vi "ASE Kalman_Experiment_FPGA.vi"() -> ()   [LabVIEW 2018]
doc: "This example demonstrates a simple analog loopback."
uses:
  <vilib>/Simulation/Scripting/Companion Diagram/SimConfigNode/SimDog.xnode
  <vilib>/Simulation/Implementation/Shared/SIMSCR Execution Mode.ctl
  <vilib>/Simulation/Scripting/Companion Diagram/SimConfigNode/_simSolvers.ctl
  <vilib>/Simulation/Scripting/Companion Diagram/SimConfigNode/SimParams.ctl
  <vilib>/Simulation/Implementation/XNodeFramework/SimXNode/SimX.xnode
  <vilib>/Simulation/SignalArithmetic/Implementation/NILVSim Gain.llb/SIM Gain (scalar).vi
  <vilib>/Simulation/ContinuousLinear/Implementation/NILVSim Transfer Function.llb/SIM Transfer Function (SISO).vi
  <vilib>/Simulation/Utility/Implementation/SIM Halt.vi
  <vilib>/Simulation/DataSources/Implementation/NILVSim Signal Generator.llb/SIM Signal Generator (scalar).vi
  <vilib>/Simulation/Nonlinear/Implementation/NILVSim Saturation.llb/SIM Saturation (scalar).vi
  <vilib>/Simulation/Nonlinear/Implementation/NILVSim RateLimiter.llb/SIM RateLimiter (scalar).vi
  <vilib>/Simulation/ContinuousLinear/Implementation/NILVSim Integrator new.llb/SIM Integrator (scalar).vi
  <vilib>/rvi/interface/nirviReadWriteControl/nirviReadWriteControl.xnode
  NiFpgaLv.dll
  <vilib>/Utility/error.llb/Error Cluster From Error Code.vi
  <vilib>/rvi/interface/Simulation/niFpgaSimulationCallBeginRW.vi
  <vilib>/rvi/errors/niLvFpgaAdjustHostInterfaceError.vi
  <vilib>/Quanser/Rapid Control Prototyping Toolkit/discrete/CL Bias Removal.vi
  <vilib>/Quanser/Rapid Control Prototyping Toolkit/discrete/_TypeSpecific/CL Bias Removal (Scalar).vi
  <vilib>/rvi/interface/nirviOpenFPGA/nirviOpenFPGA.xnode
  <vilib>/Simulation/SignalArithmetic/Implementation/NILVSim Gain.llb/SIM Gain (vector).vi
  <vilib>/Simulation/Nonlinear/Implementation/NILVSim Saturation.llb/SIM Saturation (vector).vi
  <vilib>/rvi/interface/nirviCloseFPGA/nirviCloseFPGA.xnode
  <vilib>/FPGAPlugInAG/Dynamic/niLvFpga_Close_Dynamic.vi
  <vilib>/addons/Control Design/_Stochastic Systems/NI_CD_Stochastic Systems.lvlib
  <vilib>/addons/Control Design/_Stochastic Systems/Stochastic Systems.llb/CD Construct Stochastic Model (Numeric).vi
  <vilib>/addons/Control Design/_Stochastic Systems/Stochastic Systems.llb/CD Construct Noise Model (Numeric).vi
  <vilib>/addons/Control Design/_Implementation/CD Continuous Recursive Kalman Filter.vi
  <vilib>/imath/engines/lvmath2/RunTimeEngine/Managers/WorkSpace/UID Generator.vi
  <vilib>/imath/engines/lvmath2/RunTimeEngine/LocalVariableDefStatement/MC_LocalVariableDefStatement_Display.vi
  <vilib>/imath/engines/lvmath2/RunTimeEngine/RunTimeType/NIMS_RunTimeType_From StrictType (excl LVString).vi
  <vilib>/imath/engines/lvmath2/RunTimeEngine/Managers/SymbolTable/Clear UID.vi
  <vilib>/imath/engines/lvmath2/RunTimeEngine/Managers/SymbolTable/NIMS_WorkSpace.lvlib
  <vilib>/imath/engines/lvmath2/RunTimeEngine/NodeEndStatement/NIMS_NodeEndStatement_Output.vi
  <vilib>/imath/engines/lvmath2/RunTimeEngine/ErrorHandling/NIMS_Finalize Error.vi
  <vilib>/Simulation/SignalDisplay/Implementation/NILVSim Time Waveform.llb/SIM Time Waveform (vector).vi
  FPGA Bitfiles/ActiveSuspension_FPGATarget_FPGAQ1MODULE_-QPaFzs6Ihw.lvbitx
  FPGA_Q1_MODULE.vi
  <vilib>/FPGAPlugInAG/cRIO-9068/niLvFpga_Open_cRIO-9068.vi
  <vilib>/rvi/interface/common/dynamic/niFpgaDynamicAddResources.vi
panel:
  out "Kalman Filter":waveform(dbl)[](graph)=[{"t0"=timestamp(9.964 s since 1904-01-01), "dt"=1.0, "Y"=[0.009999999999999988]}, {"t0"=timestamp(9.964 s since 1904-01-01), "dt"=1.0, "Y"=[0.008101035650175014]}, {"t0"=timestamp(9.964 s since 1904-01-01), "dt"=1.0, "Y"=[0.0033426903430059957]}]
  out "Measured value":T1(graph)={"output"=0.0096065956, "Result"=0.0090666584, "output"=0.0091514816}
  in  "R":dbl[][](array[numeric])=[[0.001, 0.0], [0.0, 0.001]] format="%#.5f"
  in  "Q":dbl[][](array[numeric])=[[0.001, 0.0, 0.0, 0.0], [0.0, 0.001, 0.0, 0.0], [0.0, 0.0, 0.001, 0.0], [0.0, 0.0, 0.0, 0.001]] format="%#.4f"
  in  "Enable Motor":bool
  in  "Setpoint Command":T2={"Amplitude (m)"=0.01, "Frequency (Hz)"=0.3} caption="Road (Bottom Plate)\nAmplitude Command (m)" {"Frequency (Hz)" min=0.0 max=0.5 step=0.009999999776482582 format="%_3f"; "Amplitude (m)" min=-10.0 max=10.0 step=0.5 format="%_3f"}
  in  "Halt?":bool
  # "Active Suspension Adaptive Control Experiment"
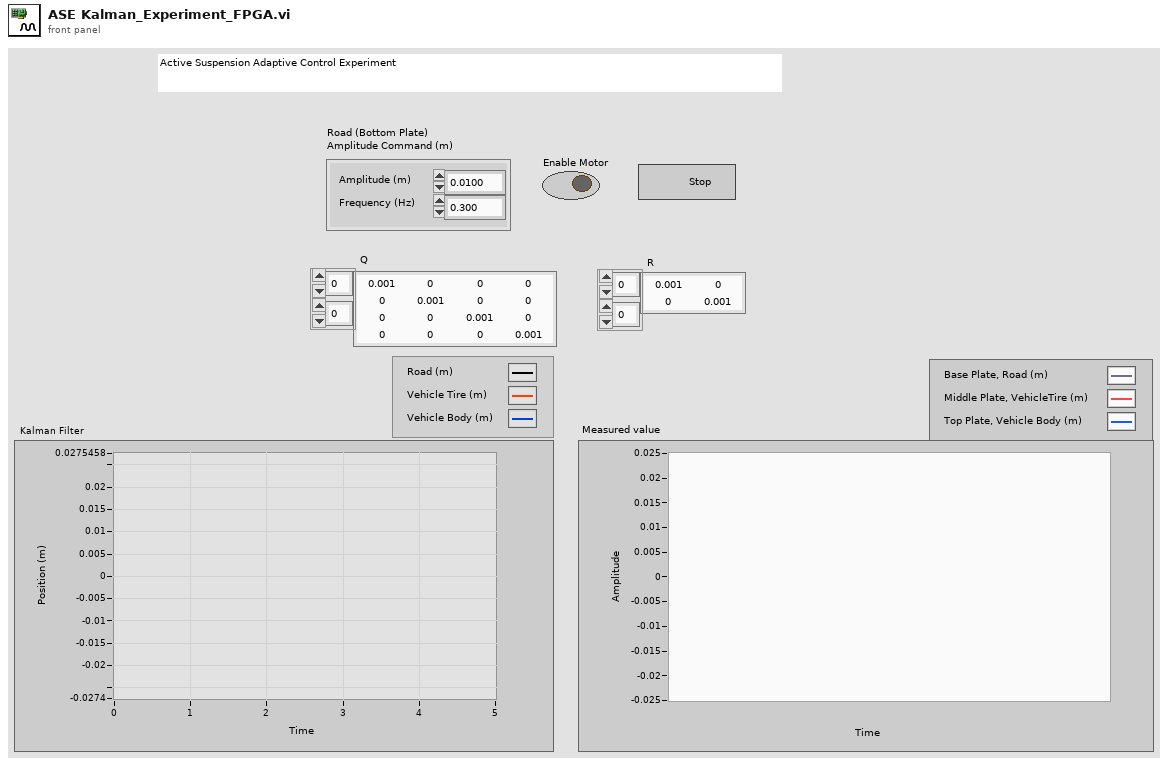
[diagram p1: front panel]
types:
  T1 = cluster{"output":dbl, "Result":dbl, "output":dbl}
  T2 = cluster{"Amplitude (m)":dbl, "Frequency (Hz)":dbl}
  T3 = typedef "SimParams.ctl" = cluster{"Initial Time (s)":dbl, "Final Time (s)":dbl, "Step Size (s)":dbl, "ODE Solver":T4, "Minimum Step Size (s)":dbl, "Maximum Step Size (s)":dbl, "Relative Tolerance":dbl, "Absolute Tolerance":dbl, "Software Timing":bool, "Initial Step Size (s)":dbl, "Automatic Fixed Step Size?":bool, "Automatic Discrete Step Size?":bool, "Discrete Step Size (s)":dbl, "Calculate using Time Step":bool, "Solver Wired?":bool, "Prev.Frm.Expected End":u64, "Prev.Frm.Actual End":u64, "Prev.Frm.Finished Late?":bool, "Prev.Iter.Expected End":u64, "Prev.Iter.Actual End":u64, "Prev.Iter.Finished Late?":bool, "Expected Iteration Start":u64, "Actual Iteration Start":u64, "Expected Frame Start":u64, "Actual Frame Start":u64, "Source Name":string, "Name":string, "Period":i64, "Deadline":i64, "Offset":i64, "Start":i64, "Priority":i32, "Timeout":i32, "Processor":i32, "Mode":enum32{"No Change", "Process missed periods, maintain original phase", "Discard missed periods, maintain original phase", "Process missed periods, ignore original phase", "Discard missed periods, ignore original phase"}, "Wakeup reason":enum32{"Normal", "Aborted", "Asynchronous wakeup", "Timing source error", "Timed loop error", "Timeout"}, "Error":errorcluster, "Source Type":string, "Secondary Source Type":string, "Global End Time":u64, "Global Start Time":u64, "Full Solver Reset":bool, "Execution Mode":T5, "Nan/Inf Check":bool, "Custom Solver Library":string, "Solver Is Variable":bool, "custom solver name":string, "Signal Collection Decimation":u32}
  T4 = typedef "_simSolvers.ctl" = enum16{"Runge-Kutta 1 (Euler)", "Runge-Kutta 2", "Runge-Kutta 3", "Runge-Kutta 4", "Runge-Kutta 23 (variable)", "Runge-Kutta 45 (variable)", "BDF (variable)", "Adams-Moulton (variable)", "Rosenbrock (variable)", "Discrete States Only", "SDIRK 4 (variable)", "Radau 5 (variable)", "Radau 9 (variable)", "Radau 13 (variable)", "Radau [Variable Order] (variable)", "Gear's Method (variable)", "Linearizer", "State Query", "Trim Eval", "Custom Solver"}
  T5 = typedef "SIMSCR Execution Mode.ctl" = enum16{"Simulate to Completion", "Single Time-Step Simulation (Fixed Step Only)"}
  T6 = typedef "NI_CD_Stochastic Systems.lvlib/cd_Stochastic State-Space Model.ctl" = cluster{"Sampling Time (s)":dbl, "G":dbl[][], "B":dbl[][], "A":dbl[][], "C":dbl[][], "D":dbl[][], "H":dbl[][]}
  T7 = typedef "NI_CD_Stochastic Systems.lvlib/cd_Second-Order Statistics Noise Model.ctl" = cluster{"Q":dbl[][], "E{w}":dbl[], "E{v}":dbl[], "R":dbl[][], "N":dbl[][]}
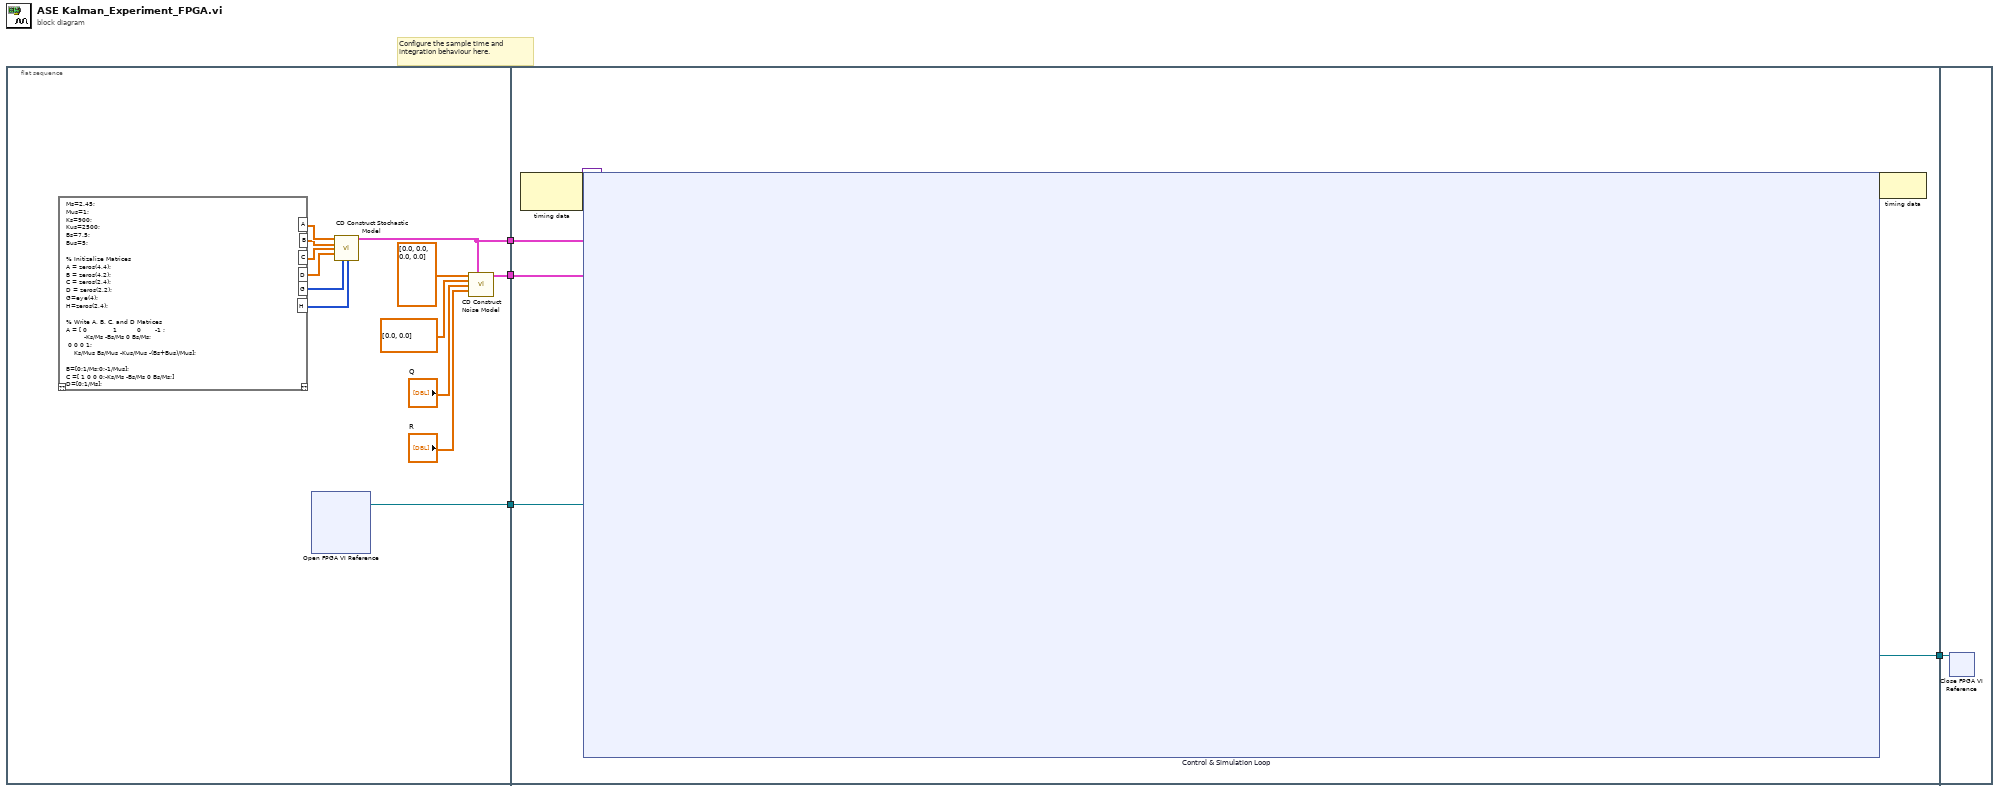
[diagram p0: block diagram]
diagram:
  # "Configure the sample time and integration behaviour here."
  n1 = flat-sequence {
    tunnel: [w17] -> w4
    tunnel: [w6] -> w2
    tunnel: [w5] -> w1
    tunnel: w4 -> [w207]
    tunnel: [w208] -> w3
    tunnel: w2 -> [w206]
    tunnel: w1 -> [w205]
    tunnel: w3 -> [w445]
    frame #0 {
      n2 = mathscript code="Ms=2.45;\nMus=1;\nKs=900;\nKus=2500;\nBs=7.5;\nBus=5;\n\n% Initizalize Matrices\nA = zeros(4,4);\nB = zeros(4,2);\nC = zeros(2,4);\nD = zeros(2,2);\nG=eye(4);\nH=zeros(2,4);\n\n% Write A, B, C, and D Matrices\nA = [ 0             1          0       -1 ; \n         -Ks/Ms -Bs/Ms 0 Bs/Ms;  \n 0 0 0 1;\n    Ks/Mus Bs/Mus -Kus/Mus -(Bs+Bus)/Mus];\n\nB=[0;1/Ms;0;-1/Mus];\nC =[ 1 0 0 0;-Ks/Ms -Bs/Ms 0 Bs/Ms;]\nD=[0;1/Ms];"() -> ("A"=w16:dbl[][], "B"=w14:dbl[][], "C"=w15:dbl[][], "D"=w13:dbl[][], "G"=w10:i32[][], "H"=w9:i32[][])  [unwired: 1 in, 1 out]
      n3 = xnode "Open FPGA VI Reference"() -> ("FPGA VI Reference Out"=w17:refnum<k20>)  [unwired: 2 in, 1 out]
      n4 = call-poly <vilib>:"CD Construct Stochastic Model.vi"("A"=w16, "B"=w14, "C"=w15, "D"=w13, "G"=w10, "H"=w9) -> ("Stochastic State-Space Model"=w6:T6)  [unwired: 2 in, 7 out]
      n5 = call-poly <vilib>:"CD Construct Noise Model.vi"("E{w}"=dbl[] [0.0, 0.0, 0.0, 0.0], "Stochastic State-Space Model"=w6, "E{v}"=dbl[] [0.0, 0.0], "Q"="Q", "R"="R") -> ("Second-Order Statistics Noise Model out"=w5:T7)  [unwired: 9 in, 1 out]
    }
    frame #1 {
      n6 = node-c288() -> (w210:variant)  [unwired: 2 in]
      n7 = node-c254 "Control & Simulation Loop"(w210, w207, w206, w205) -> (w209:variant, w208:refnum<k20>)
      n8 = node-c288(w209) -> ()  [unwired: 1 out]
    }
    frame #2 {
      n9 = xnode "Close FPGA VI Reference"("FPGA VI Reference In"=w445) -> ()  [unwired: 1 in, 1 out]
    }
  }
